vi "CSM - Revert Arguments-Safe String.vi"(2 "Safe Argument String":string="eaasdf->fqwvrf", 4 "Force Convert (F)":bool) -> (7 "Origin Argument String":string)   [LabVIEW 2017, in "Communicable State Machine.lvlib"]
doc: "Converts the %Hex format CSM keywords in the safe string argument back to the original format.\n\n- When <b>Force Convert (F)</b> is FALSE, conversion is performed only if the argument type tag is `SAFESTR`.\n- When <b>Force Convert (F)</b> is TRUE, conversion is performed regardless of the argument type tag.\n\n\n> [!NOTE] <b>CSM Message Keywords</b>\n>\n> The following are CSM message keywords: `->`, `->|`, `-@`, `-&`, `<-`, `\\r`, `\\n`, `//`, `>>`, `>>>`, `>>>>`, `;`, `,`.\n\n\n> [!NOTE] <b>CSM Safe String Argument</b>\n>\n> To pass arbitrary strings in CSM arguments without disrupting message parsing, CSM has a built-in Safe-String encoding/decoding scheme. The argument type string is SAFESTR. The conversion process is as follows:\n> 1. Replace `%` in the input string with `%25`.\n> 2. Scan the string. If any CSM keywords, such as `->`, `;`, `\\r` appear, replace them with `%Hex` escape sequences.\n> 3. Obtain the argument in the form `<SAFESTR> escaped string`, which can be safely embedded in the state string without disrupting CSM message parsing.\n> Decoding is the reverse process: the `%Hex` escape sequences of CSM keywords are converted back first, then `%25` is converted back to `%`.\n\n\n<b>Reference Example</b>: `[CSM-Example]\\0. Base Concepts\\4.3 Arguments - Safe Arguments if it contains key words of CSM.vi`.\n\n-- <b>Controls</b> --\n- <b>Safe Argument String</b>: Safe string argument.\n- <b>Force Convert (F)</b>: Force conversion, even if the argument type tag is not `SAFESTR`.\n\n-- <b>Indicators</b> --\n- <b>Origin Argument String</b>: String argument."
uses:
  Communicable State Machine.lvlib
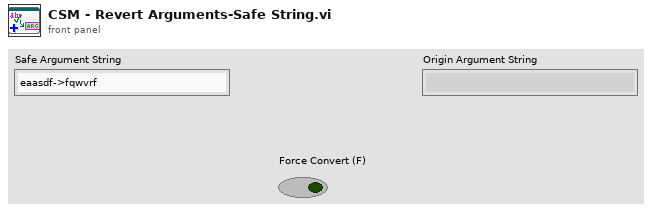
[diagram p1: front panel]
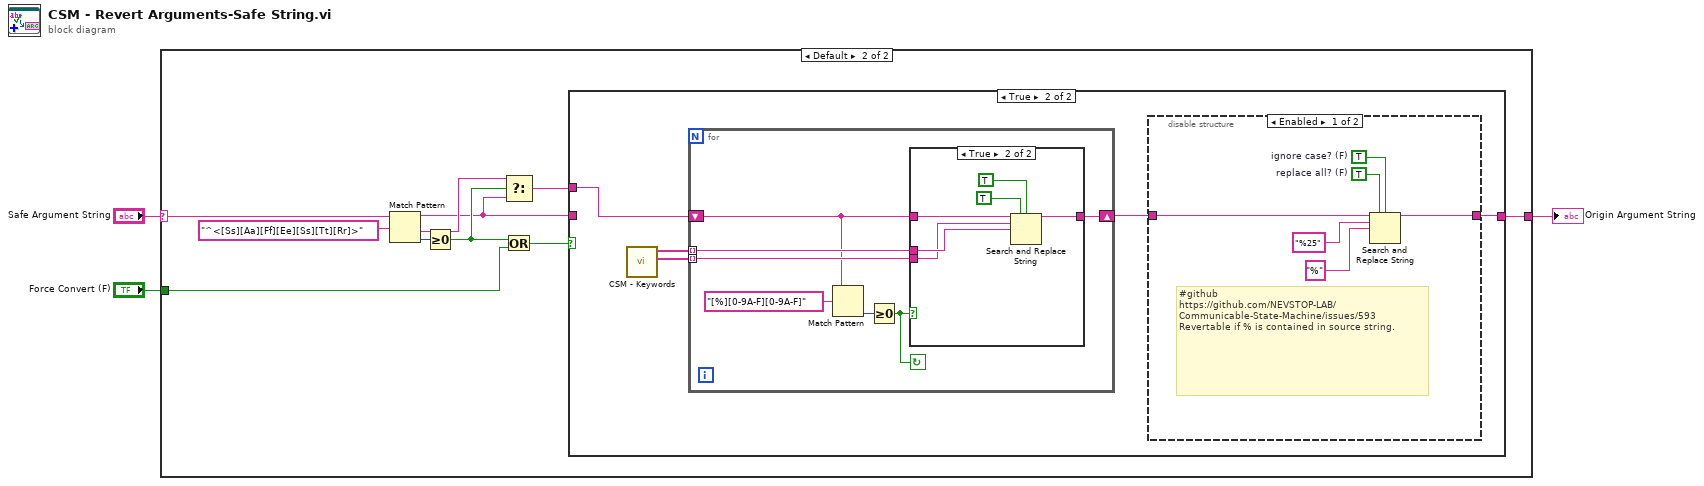
[diagram p0: block diagram]
diagram:
  n1 = case shown="Default" "Safe Argument String" {
    selector: "Safe Argument String" -> [w4 w11]
    tunnel: [w4 w14] -> w2
    tunnel: "Force Convert (F)" -> [_ w9]
    frame "" {
    }
    frame Default {
      n2 = Match Pattern(string=w11, regular expression="^<[Ss][Aa][Ff][Ee][Ss][Tt][Rr]>") -> (before substring=w6:string, after substring=w7:string, offset past match=w12:i32)  [unwired: 1 in, 1 out]
      n3 = Greater Or Equal To 0?(x=w12) -> (x >= 0?=w8:bool)
      n4 = Select(t=w7, s=w8, f=w6) -> (s? t:f=w5:string)
      n5 = Or(x=w8, y=w9) -> (x .or. y?=w10:bool)
      n6 = case shown="True" w10 {
        tunnel: [w15 w16] -> w14
        tunnel: w6 -> [w15 _]
        tunnel: w5 -> [_ w18]
        frame False {
        }
        frame True {
          n7 = call "CSM - Keywords.vi"() -> ("Keywords (%Hex Format)"=w20:string[], "Keywords"=w19:string[])  [unwired: 10 in]
          n8 = for {
            shift-right: [w34] -> w17
            shift-left: w18 -> [w31]
            tunnel: w19 -> [w33] mode=indexing
            tunnel: w20 -> [w32] mode=indexing
            stop <- w28 continue-if-true
            n9 = Match Pattern(string=w31, regular expression="[%][0-9A-F][0-9A-F]") -> (offset past match=w29:i32)  [unwired: 1 in, 3 out]
            n10 = Greater Or Equal To 0?(x=w29) -> (x >= 0?=w28:bool)
            n11 = case shown="True" w28 {
              tunnel: [w35 w40] -> w34
              tunnel: w33 -> [_ w39]
              tunnel: w32 -> [_ w38]
              tunnel: w31 -> [w35 w37]
              frame False {
              }
              frame True {
                n12 = Search and Replace String(replace all?=TRUE ("replace all? (F)"), case sensitive?=TRUE ("ignore case? (F)"), input string=w37, search string=w38, replace string=w39) -> (result string=w40:string)  [unwired: 3 in, 3 out]
              }
            }
          }
          n13 = disable-structure shown="Enabled" {
            disable-tunnel: w17 -> [w22 w27]
            disable-tunnel: [w21 w27] -> w16
            frame Enabled {
              w25 = TRUE  # ignore case? (F)
              w26 = TRUE  # replace all? (F)
              # "#github \nhttps://github.com/NEVSTOP-LAB/Communicable-State-Machine/issues/593\nRevertable if % is contained in source string."
              n14 = Search and Replace String(replace all?=w26, case sensitive?=w25, input string=w22, search string="%25", replace string="%" ("search string")) -> (result string=w21:string)  [unwired: 3 in, 3 out]
            }
            frame Disabled {
            }
          }
        }
      }
    }
  }
  "Origin Argument String" <- w2
